vi "Write NChanNSamp error check (SubVI).vi"(7 "Analog output in":refnum<class "Analog output.lvclass">, 8 "error in (no error)":errorcluster, 11 "data":sgl[][](array[numeric])) -> (0 "error out":errorcluster)   [LabVIEW 2009, in "MicroDAQ.lvlib" / "Analog output.lvclass"]
doc: "Writes waveform to all channels."
uses:
  <instrlib>/MicroDAQ/Channel/Analog Output/Analog output.lvclass
  <instrlib>/MicroDAQ/Channel/Analog Output/Analog output.lvclass/Analog output.ctl
  <instrlib>/MicroDAQ/MicroDAQ.lvlib
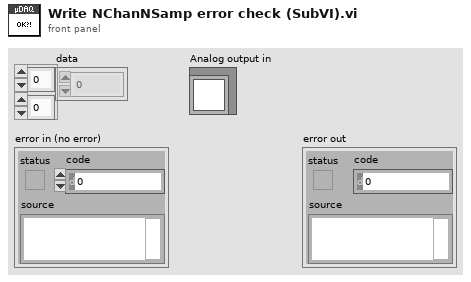
[diagram p1: front panel]
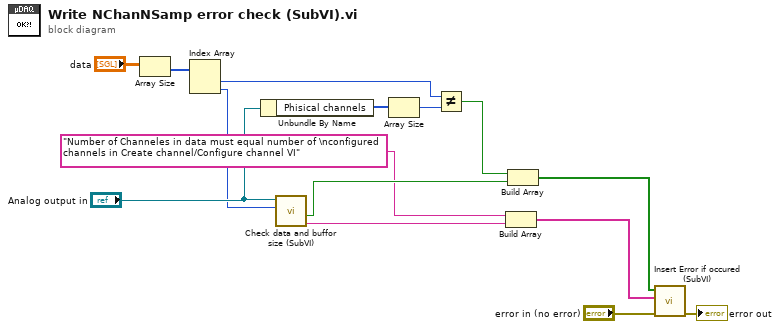
[diagram p0: block diagram]
diagram:
  n1 = Array Size(array="data") -> (size(s)=w8:i32[])
  n2 = Index Array(array=w8) -> (element #1=w2:i32, element #2=w1:i32)  [unwired: 2 in]
  n3 = Unbundle By Name("Analog output in") -> ("Phisical channels"=w6:u8[])
  n4 = call <instrlib>:"Check data and buffor size (SubVI).vi"("data size"=w1, "Analog output in"="Analog output in") -> ("Error message"=w12:string, "Error?"=w13:bool)  [unwired: 8 in]
  n5 = Array Size(array=w6) -> (size(s)=w5:i32)
  n6 = Not Equal?(x=w2, y=w5) -> (x != y?=w4:bool)
  n7 = Build Array("Number of Channeles in data must equal number of \nconfigured channels in Create channel/Configure channel VI" ("element"), w12) -> (w10:string[])
  n8 = Build Array(w4, w13) -> (w11:bool[])
  n9 = call <instrlib>:"Insert Error if occured (SubVI).vi"("error in (no error)"="error in (no error)", "Error messages"=w10, "Error conditionals"=w11) -> ("error out"=→"error out":errorcluster)  [unwired: 8 in]
